vi "temperature-measurement.vi"(5 "Enter RH [%]":dbl format="%#_13g", 7 "Enter temp. [°C]":dbl format="%#_13g", 8 "error in (no error)":errorcluster, 9 "Instrument":enum16{"AG34401A", "Arduino", "Manually"}(ring), 10 "Action":enum16{"initialize", "measure", "close"}(ring), 11 "Address (for temperature)":refnum<visa-resource-name>="GPIB0::22::INSTR") -> (0 "error out":errorcluster, 1 "RH [%]":dbl, 2 "T [°C]":dbl, 3 "VISA resource name out":refnum<visa-resource-name>)   [LabVIEW 2018]
uses:
  <instrlib>/Agilent 34401/Public/Data/Read (Single Point).vi
  <vilib>/express/express shared/transition.llb/Dynamic To Waveform Array.vi
  <vilib>/express/express arith-compare/Formula/Block/exnFormulaBlock how many pts in the wave.vi
  <vilib>/express/express shared/ex_Modify Signal Name.vi
  <vilib>/express/express shared/transition.llb/Waveform Array To Dynamic.vi
  <vilib>/express/express arith-compare/Formula/XNode/ExpressFormulaBlockNode.xnode
  <instrlib>/Agilent 34401/Agilent 34401.lvlib
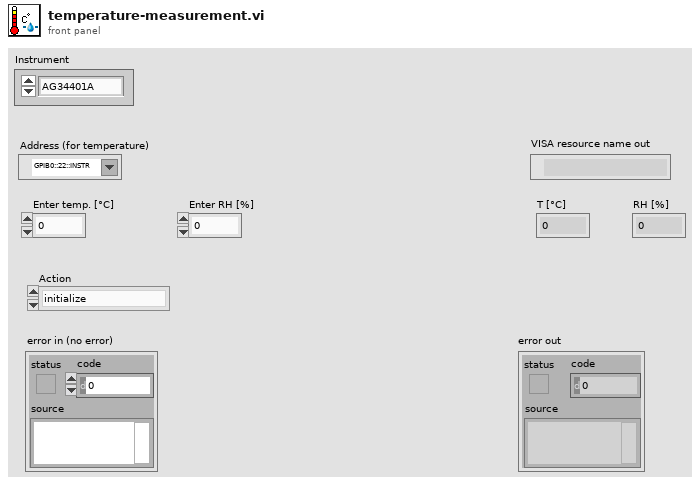
[diagram p1: front panel]
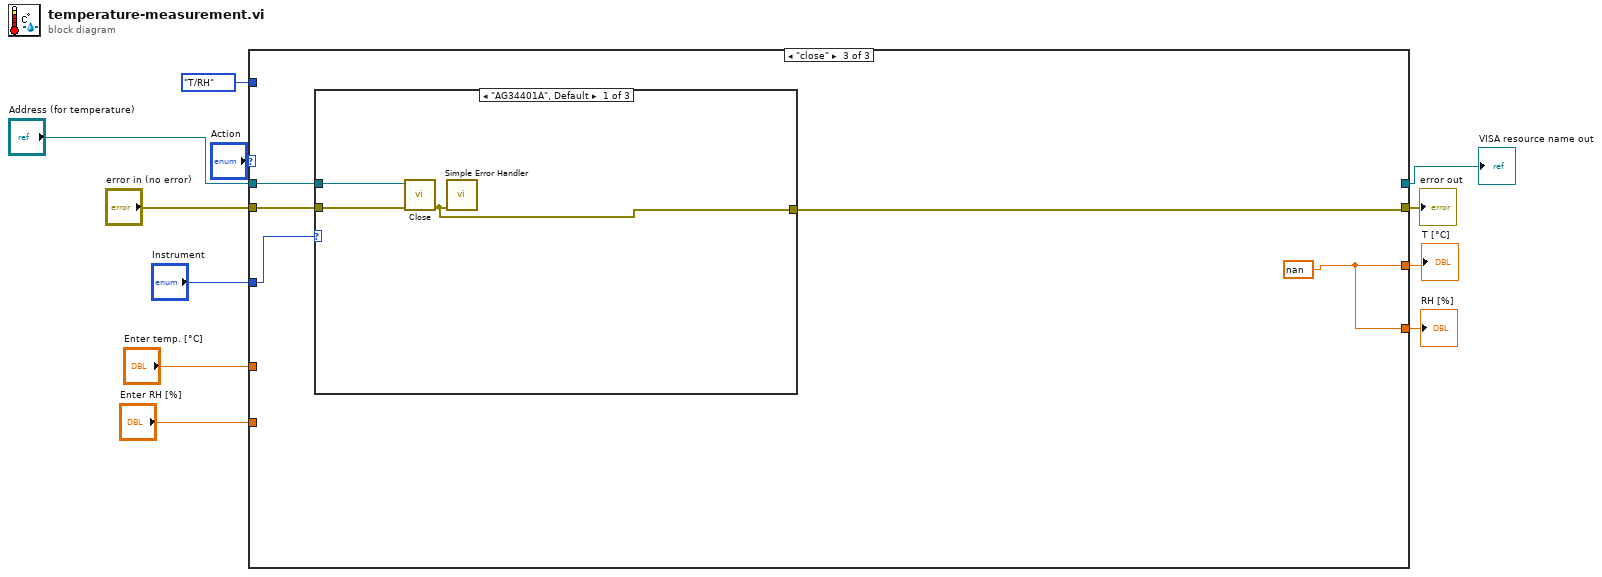
[diagram p0: block diagram]
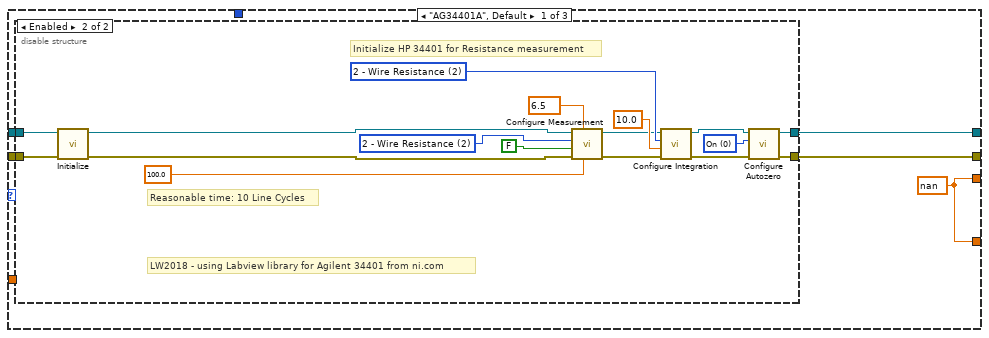
[diagram p3: hidden frame]
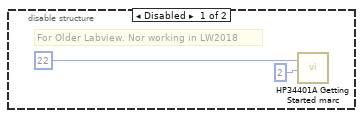
[diagram p4: hidden frame]
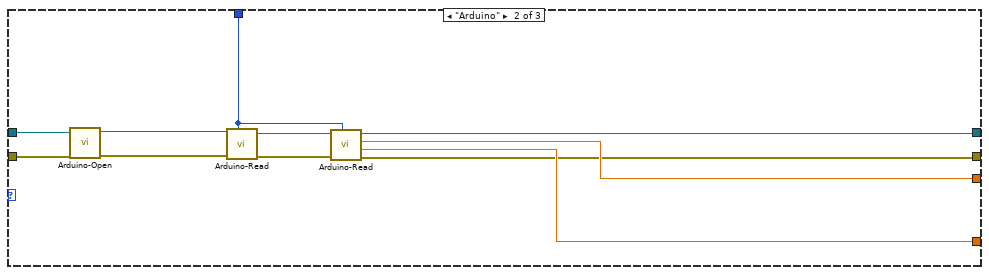
[diagram p5: hidden frame]
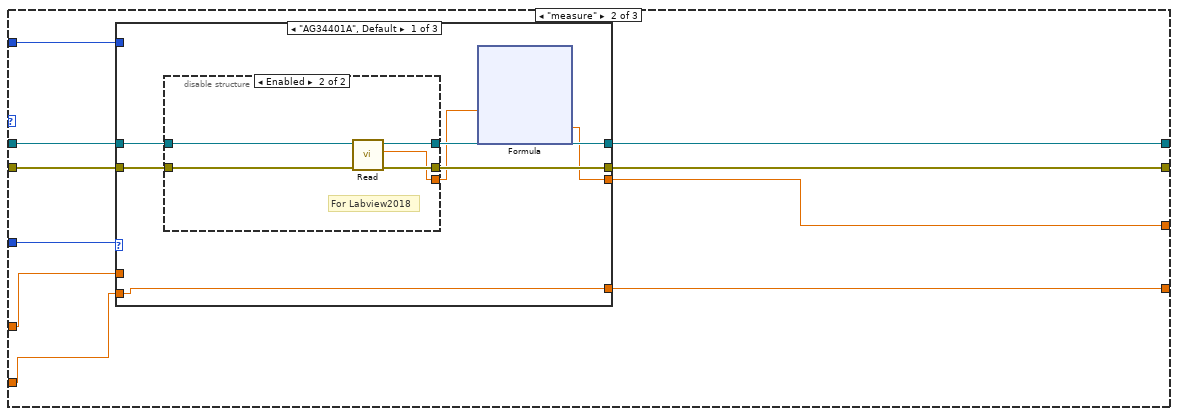
[diagram p6: hidden frame]
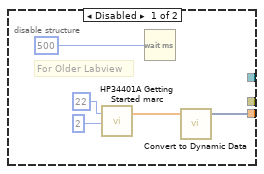
[diagram p7: hidden frame]
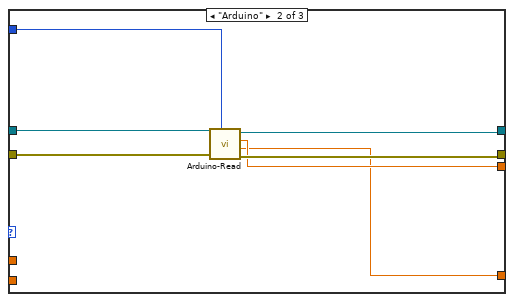
[diagram p8: hidden frame]
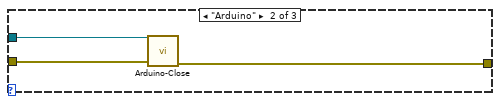
[diagram p10: hidden frame]
diagram:
  n1 = case shown="\"close\"" "Action" {
    tunnel: "Address (for temperature)" -> [w21 w70 w242]
    tunnel: "error in (no error)" -> [w20 w69 w241]
    tunnel: [w19 w68 _] -> w8
    tunnel: [w18 w67 w239] -> w7
    tunnel: [w15 w66 w238] -> w6
    tunnel: "Instrument" -> [w17 w65 w240]
    tunnel: enum16{"T/RH", "Interlock", "Edgesense"}."T/RH" ("Arduino function") -> [w16 w64 _]
    tunnel: [w14 w63 w238] -> w3
    tunnel: "Enter temp. [°C]" -> [w13 w61 _]
    tunnel: "Enter RH [%]" -> [w12 w62 _]
    frame "initialize", Default {
      n2 = case shown="\"Manually\"" w17 {
        tunnel: w21 -> [w26 w56 w60]
        tunnel: w20 -> [w25 w55 w59]
        tunnel: [w24 w46 w60] -> w19
        tunnel: [w23 w47 w59] -> w18
        tunnel: w16 -> [_ w50 _]
        tunnel: [w22 w49 w58] -> w15
        tunnel: [w22 w48 w57] -> w14
        tunnel: w13 -> [_ _ w58]
        tunnel: w12 -> [_ _ w57]
        frame "AG34401A", Default {
          w22 = nan
          n3 = disable-structure shown="Enabled" {
            disable-tunnel: w26 -> [_ w32]
            disable-tunnel: w25 -> [_ w31]
            disable-tunnel: [_ w30] -> w24
            disable-tunnel: [_ w29] -> w23
            frame Disabled {
              # "For Older Labview. Nor working in LW2018"
              n4 = call "HP34401A Getting Started marc.vi"("Address/Port (22)"=22, "Function (0:V DC)"=2) -> ()  [unwired: 16 in, 2 out]
            }
            frame Enabled {
              w45 = 10.0 items=["0.001"=0.001, "0.002"=0.002, "0.006"=0.006, "0.02"=0.02, "0.06"=0.06, "0.2"=0.2, "1"=1.0, "10"=10.0, "100"=100.0] ("Integration Time (1 PLCs)")
              w44 = u16 2 items=["DC Voltage", "AC Voltage", "2 - Wire Resistance", "4 - Wire Resistance", "DC Current", "AC Current", "Frequency", "Period", "Continuity", "Diode Checking", "VDC:VDC Ratio", "Temperature", "Capacitance"] ("Function (0: DC Voltage)")
              w37 = u16 0 items=["On", "Off", "Once"] ("Autozero  (0: On)")
              w36 = 6.5 items=["4.5"=4.5, "5.5"=5.5, "6.5"=6.5] ("Manual Resolution (5.5 Digits)")
              w35 = u16 2 items=["DC Voltage", "AC Voltage", "2 - Wire Resistance", "4 - Wire Resistance", "DC Current", "AC Current", "Frequency", "Period", "Continuity", "Diode Checking", "VDC:VDC Ratio", "Temperature", "Capacitance"] ("Function (0: DC Voltage)")
              # "LW2018 - using Labview library for Agilent 34401 from ni.com"
              # "Reasonable time: 10 Line Cycles"
              # "Initialize HP 34401 for Resistance measurement"
              n5 = call <instrlib>:"Initialize.vi"("error in (no error)"=w31, "VISA resource name"=w32) -> ("error out"=w34:errorcluster, "VISA resource name out"=w33:refnum<visa-resource-name>)  [unwired: 8 in]
              n6 = call <instrlib>:"Configure Measurement.vi"("Manual Range (1.00)"=100.0, "Manual Resolution (5.5 Digits)"=w36, "error in (no error)"=w34, "Enable Auto Range (T: Enable)"=FALSE, "Function (0: DC Voltage)"=w35, "VISA resource name"=w33) -> ("error out"=w41:errorcluster, "VISA resource name out"=w40:refnum<visa-resource-name>)  [unwired: 4 in]
              n7 = call <instrlib>:"Configure Integration.vi"("error in (no error)"=w41, "Integration Time (1 PLCs)"=w45, "Function (0: DC Voltage)"=w44, "VISA resource name"=w40) -> ("error out"=w42:errorcluster, "VISA resource name out"=w43:refnum<visa-resource-name>)  [unwired: 6 in]
              n8 = call <instrlib>:"Configure Autozero.vi"("error in (no error)"=w42, "Autozero  (0: On)"=w37, "VISA resource name"=w43) -> ("error out"=w29:errorcluster, "VISA resource name out"=w30:refnum<visa-resource-name>)  [unwired: 7 in]
            }
          }
        }
        frame "Arduino" {
          n9 = call "Arduino-Open.vi"("error in (no error)"=w55, "Visa Resource"=w56) -> ("error out"=w53:errorcluster, "VISA resource name out"=w54:refnum<visa-resource-name>)  [unwired: 7 in, 1 out]
          n10 = call "Arduino-Read.vi"("Arduino function"=w50, "error in (no error)"=w53, "VISA resource name"=w54) -> ("error out"=w52:errorcluster, "VISA resource name out"=w51:refnum<visa-resource-name>)  [unwired: 3 in, 4 out]
          n11 = call "Arduino-Read.vi"("Arduino function"=w50, "error in (no error)"=w52, "VISA resource name"=w51) -> ("error out"=w47:errorcluster, "rel. Humidity [%]"=w48:dbl, "Temperature [°C]"=w49:dbl, "VISA resource name out"=w46:refnum<visa-resource-name>)  [unwired: 3 in, 2 out]
        }
        frame "Manually" {
        }
      }
    }
    frame "measure" {
      n12 = case shown="\"AG34401A\", Default" w65 {
        tunnel: w70 -> [w77 w232 w234]
        tunnel: w69 -> [w76 w231 w235]
        tunnel: [w75 w230 w234] -> w68
        tunnel: [w74 w229 w235] -> w67
        tunnel: [w71 w228 w236] -> w66
        tunnel: w64 -> [_ w233 _]
        tunnel: [w73 w227 w237] -> w63
        tunnel: w62 -> [w73 _ w237]
        tunnel: w61 -> [_ _ w236]
        frame "AG34401A", Default {
          n13 = disable-structure shown="Enabled" {
            disable-tunnel: [w218 w222] -> w72
            disable-tunnel: w77 -> [_ w226]
            disable-tunnel: w76 -> [_ w225]
            disable-tunnel: [_ w224] -> w75
            disable-tunnel: [_ w223] -> w74
            frame Disabled {
              # "For Older Labview"
              n14 = call "HP34401A Getting Started marc.vi"("Address/Port (22)"=22, "Function (0:V DC)"=2) -> ("Measurements"=w219:dbl[])  [unwired: 16 in, 1 out]
              n15 = Wait (ms)(milliseconds to wait=500) -> ()  [unwired: 1 out]
              n16 = call "Convert to Dynamic Data"("Array"=w219) -> ("Dynamic Data Type"=w218:dynamicdata)  [unwired: 3 in]
            }
            frame Enabled {
              # "For Labview2018"
              n17 = call-poly <instrlib>:"Read.vi"("error in (no error)"=w225, "VISA resource name"=w226) -> ("error out"=w223:errorcluster, "Measurement"=w222:dbl, "VISA resource name out"=w224:refnum<visa-resource-name>)  [unwired: 7 in]
            }
          }
          n18 = xnode "Formula"("X1"=w72) -> ("Result"=w71:dbl)  [unwired: 1 in, 1 out]
        }
        frame "Arduino" {
          n19 = call "Arduino-Read.vi"("Arduino function"=w233, "error in (no error)"=w231, "VISA resource name"=w232) -> ("error out"=w229:errorcluster, "rel. Humidity [%]"=w227:dbl, "Temperature [°C]"=w228:dbl, "VISA resource name out"=w230:refnum<visa-resource-name>)  [unwired: 3 in, 2 out]
        }
        frame "Manually" {
        }
      }
    }
    frame "close" {
      w238 = nan
      n20 = case shown="\"AG34401A\", Default" w240 {
        tunnel: w242 -> [w245 w247 _]
        tunnel: w241 -> [w244 w248 w249]
        tunnel: [w243 w246 w249] -> w239
        frame "AG34401A", Default {
          n21 = call <instrlib>:"Close.vi"("error in (no error)"=w244, "VISA resource name"=w245) -> ("error out"=w243:errorcluster)  [unwired: 9 in]
          n22 = call <vilib>:"Simple Error Handler.vi"("error in (no error)"=w243) -> ()  [unwired: 4 in, 5 out]
        }
        frame "Arduino" {
          n23 = call "Arduino-Close.vi"("error in (no error)"=w248, "VISA resource name"=w247) -> ("error out"=w246:errorcluster)  [unwired: 9 in]
        }
        frame "Manually" {
        }
      }
    }
  }
  "VISA resource name out" <- w8
  "error out" <- w7
  "T [°C]" <- w6
  "RH [%]" <- w3
